vi "StepperGetVelocity.vi"(0 "error in (no error)":errorcluster, 3 "Device In":u64) -> (7 "error out":errorcluster, 9 "Velocity":dbl, 10 "Device Out":u64)   [LabVIEW 2012, in "Phidget Stepper.lvlib"]
doc: "${Velocity:Header}"
uses:
  <instrlib>/Phidgets/Phidget Stepper/Phidget Stepper.lvlib
  <instrlib>/Phidgets/Phidget Common/Phidget Common.lvlib
  phidget22.dll
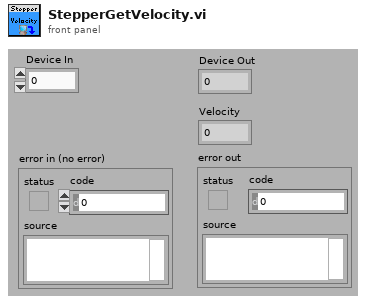
[diagram p1: front panel]
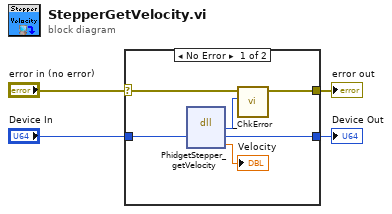
[diagram p0: block diagram]
diagram:
  n1 = case shown="No Error" "error in (no error)" {
    selector: "error in (no error)" -> [w6 w12]
    tunnel: [w5 w12] -> w3
    tunnel: "Device In" -> [w9 w11]
    tunnel: [w8 w11] -> w1
    frame No Error {
      n2 = dll-call lib="phidget22.*" fn="PhidgetStepper_getVelocity"("phid"=w9) -> ("return type"=w7:i32, "phid"=w8:u64, "temperature"=→"Velocity":dbl)  [unwired: 4 in, 2 out]
      n3 = call <instrlib>:"_ChkError.vi"("Return Code"=w7, "error in (no error)"=w6) -> ("error out"=w5:errorcluster)  [unwired: 9 in]
    }
    frame Error {
    }
  }
  "error out" <- w3
  "Device Out" <- w1
